vi "Word_Open_Document.vi"(4 "error in":errorcluster, 6 "document path":path, 7 "word application":refnum<k7>) -> (0 "error out":errorcluster, 3 "references":T1)   [LabVIEW 2010, in "NI_ReportGenerationToolkit.lvlib"]
uses:
  <vilib>/addons/_office/NI_ReportGenerationToolkit.lvlib
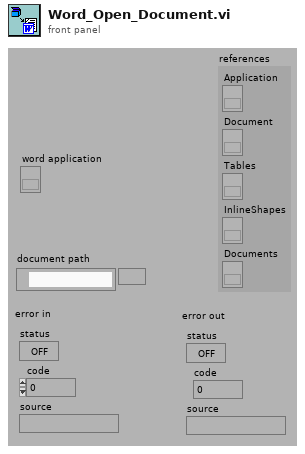
[diagram p1: front panel]
types:
  T1 = cluster{"Application":refnum<k7>, "Document":refnum<k7>, "Tables":refnum<k7>, "InlineShapes":refnum<k7>, "Documents":refnum<k7>}
  T2 = cluster{"word application":refnum<k7>, "Open":refnum<k7>, "Tables":refnum<k7>, "InlineShapes":refnum<k7>, "Documents":refnum<k7>}
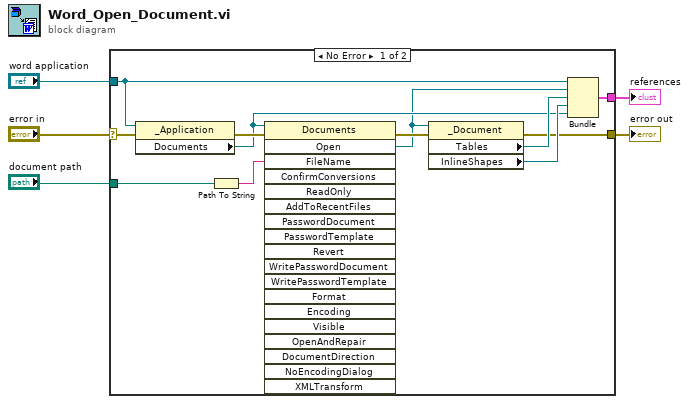
[diagram p0: block diagram]
diagram:
  n1 = case shown="No Error" "error in" {
    selector: "error in" -> [w9 w18]
    tunnel: "word application" -> [w8 _]
    tunnel: "document path" -> [w14 _]
    tunnel: [w12 _] -> w3
    tunnel: [w11 w18] -> w2
    frame No Error {
      n2 = property class="_Application"(reference=w8, error in=w9) -> (error out=w17:errorcluster, "Documents"=w7:refnum<k7>)  [unwired: 1 out]
      n3 = Path To String(path=w14) -> (string=w13:string)
      n4 = invoke class="Documents" method="Open"(reference=w7, error in=w17, "FileName"=w13) -> (error out=w10:errorcluster, "Open"=w6:refnum<k7>)  [unwired: 16 in, 17 out]
      n5 = property class="_Document"(reference=w6, error in=w10) -> (error out=w11:errorcluster, "Tables"=w16:refnum<k7>, "InlineShapes"=w15:refnum<k7>)  [unwired: 1 out]
      n6 = Bundle("word application"=w8, "Open"=w6, "Tables"=w16, "InlineShapes"=w15, "Documents"=w7) -> (w12:T2)  [unwired: 1 in]
    }
    frame Error {
    }
  }
  "error out" <- w2
  "references" <- w3
